vi "_BlankServer.vi"() -> ()   [LabVIEW 2010]
doc: "Template server that runs individual ros topics, services, etc. This is cloned for each topic being run."
uses:
  <userlib>/ROSforLV_0.1/ROS/Code/SubVIs/_ROSControl.ctl
  <userlib>/ROSforLV_0.1/ROS/Code/SubVIs/_ROSDirection.ctl
  <userlib>/ROSforLV_0.1/ROS/Code/_ROSDefinition.vi
panel:
  out "str to write":string
  out "Status":T1(ring) caption="Connected?"
  out "Specs":T3={"Server"="", "Node"="/labview", "Server Port"=5000, "URI (Subsc)"="", "Direction"=enum."Node"}
  out "Service Reply":string
  out "unregister":string="<?xml version='1.0'?>\n<methodResponse>\n<params>\n<param>\n<value><array><data>\n<value><int>1</int></value>\n<value><string>Registered [/labview] as publisher of [/robot/head/command_head_nod]</string></value>\n<value><array><data>\n<value><string>http://tuftsBaxter.local:56995/</string></value>\n</data></array></value>\n</data></array></value>\n</param>\n</params>\n</methodResponse>\n"
  out "Requests":T4(array[cluster])
  out "Last Reply":string
  in  "stop":bool
  out "error out":errorcluster
  out "Connections":T5(array[cluster])
  in  "Baxter":T6
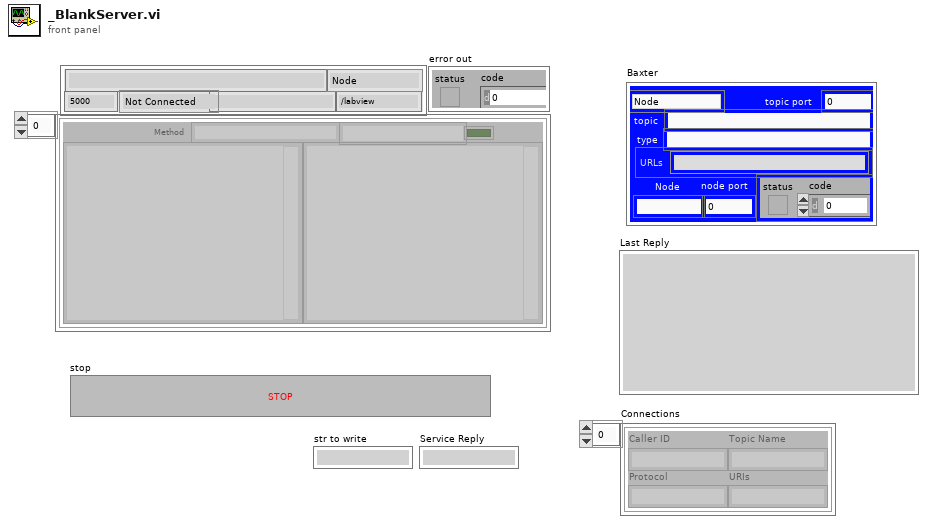
[diagram p1: front panel]
types:
  T1 = enum16{"Not Connected", "Registered", "Connected"}
  T2 = typedef "_ROSDirection.ctl" = enum16{"Node", "Publisher", "Subscriber", "Service Client"}
  T3 = cluster{"Server":string, "Node":string, "Server Port":u32, "URI (Subsc)":string, "Direction":T2}
  T4 = cluster{"First":string, "Second":string, "Method":string, "success":bool, "Dir1":string, "Dir2":string, "time":string}[]
  T5 = cluster{"Caller ID":string, "Topic Name":string, "Protocol":string, "URIs":string}[]
  T6 = typedef "_ROSControl.ctl" = cluster{"topic port":u16, "Node":string, "topic":string, "type":string, "node port":u32, "error ":errorcluster, "Direction":T2, "APIs":string[]}
  T7 = cluster{"data out":string, "data out 2":string, "data out 3":string, "Success?":bool, "data out 4":string, "data out 5":string, "time":string}[]
  T8 = cluster{"Code":i32, "Status Message":string, "APIs":string[]}
  T9 = cluster{"Server":string, "Node":string, "Server Port":u32, "URI (Subsc)":string, "connection":refnum<k5>, "Direction":T2}
  T10 = cluster{"Caller ID":string, "Topic Name":string, "Protocol":string, "URIs":string}
  T11 = cluster{string, "data out":string, "Node":string, bool, string, string, "Current Time":string}
  T12 = cluster{"str to write":string, string, string, bool, string, string, "Current Time":string}
  T13 = cluster{"Protocol":string, "Code":i32, "IP":string, "Port":i32}
  T14 = cluster{"Node":string, "topic":string, "topic":string, "topic":string}
  T15 = cluster{"Code":i8, "statusMessage":string, "APIs":string[]}
  T16 = cluster{string, string, string, bool, string, string, "Current Time":string}
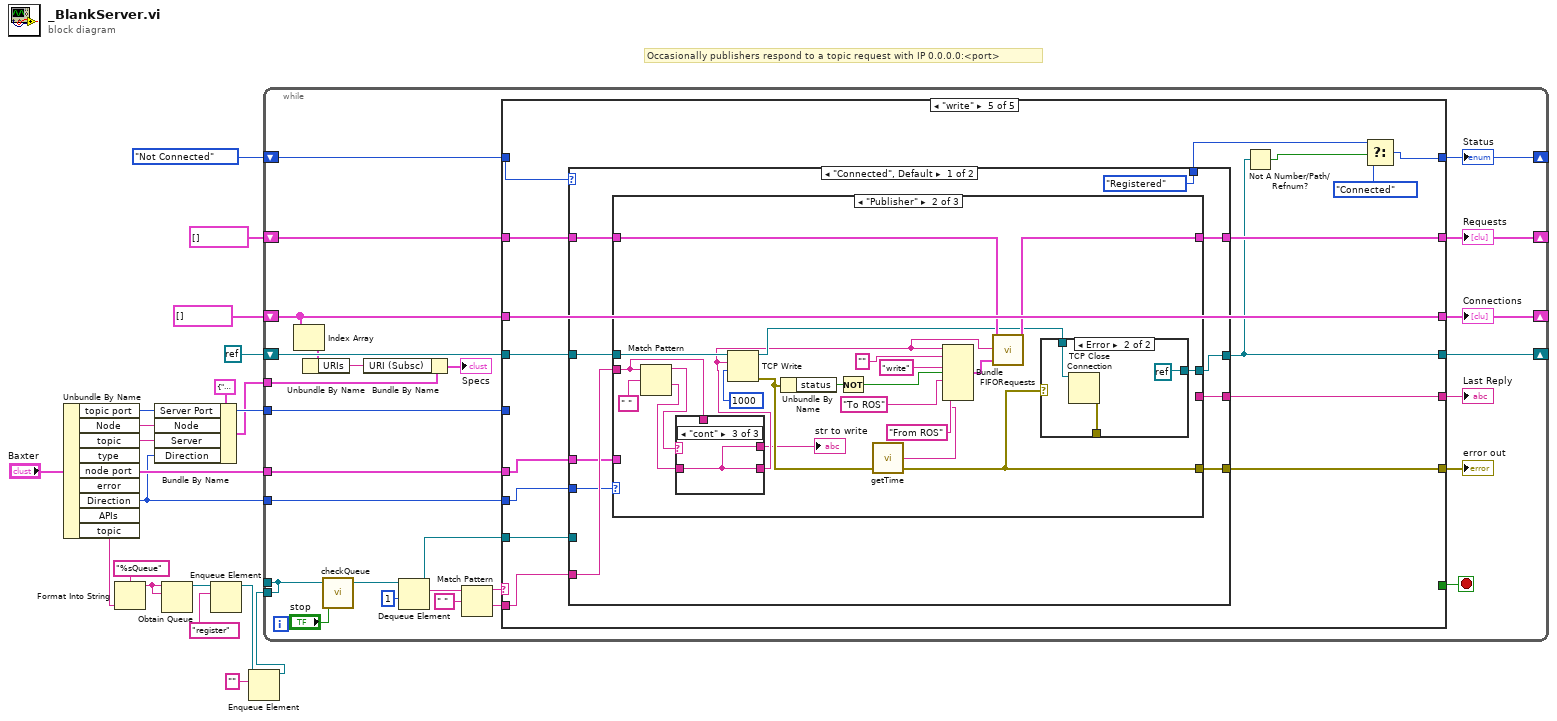
[diagram p0: block diagram]
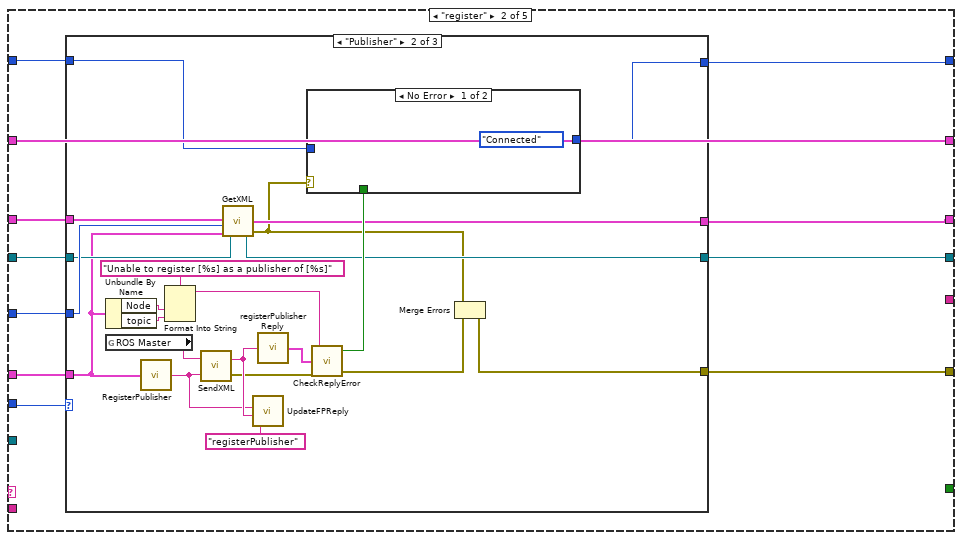
[diagram p3: hidden frame]
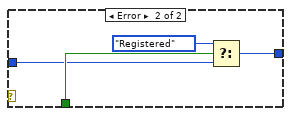
[diagram p5: hidden frame]
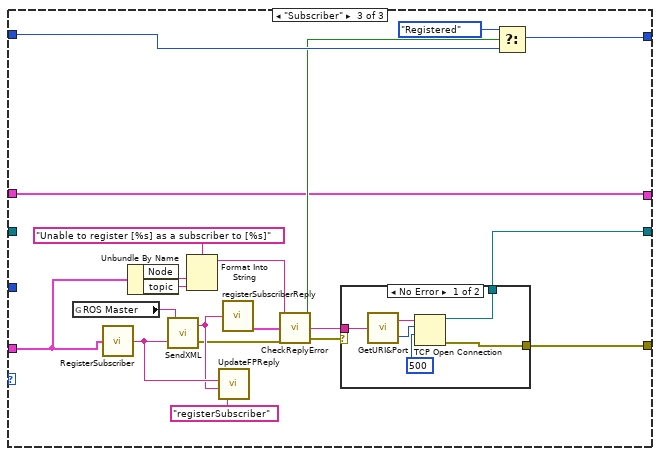
[diagram p6: hidden frame]
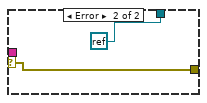
[diagram p7: hidden frame]
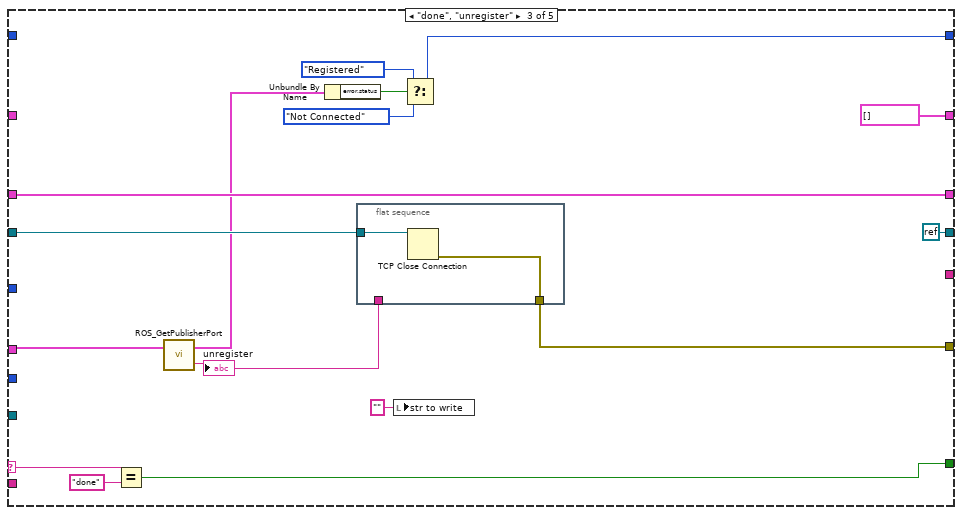
[diagram p8: hidden frame]
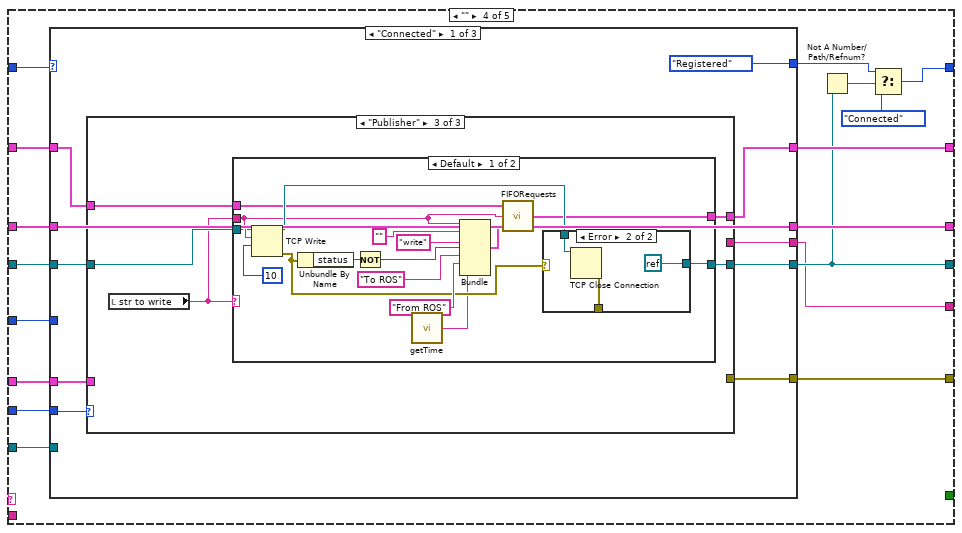
[diagram p9: hidden frame]
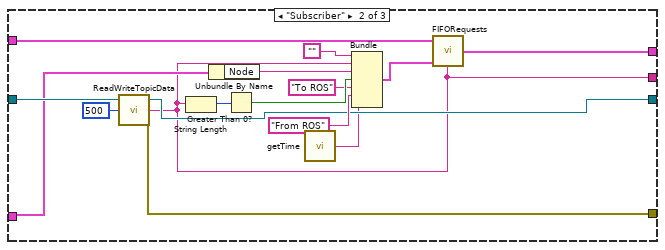
[diagram p11: hidden frame]
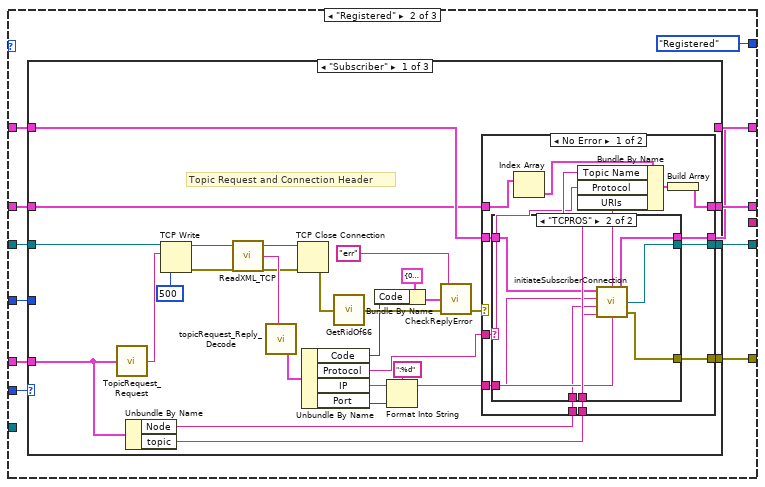
[diagram p14: hidden frame]
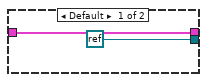
[diagram p15: hidden frame]
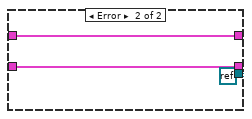
[diagram p16: hidden frame]
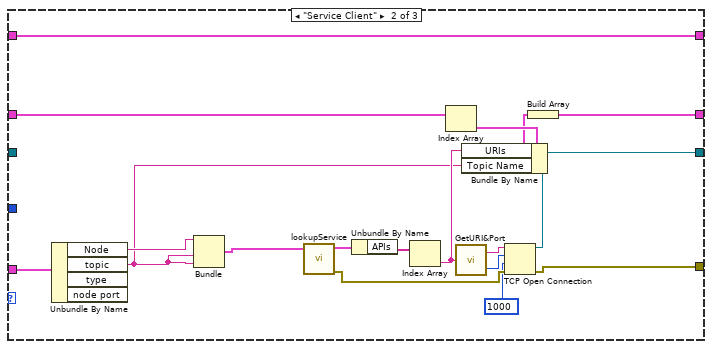
[diagram p17: hidden frame]
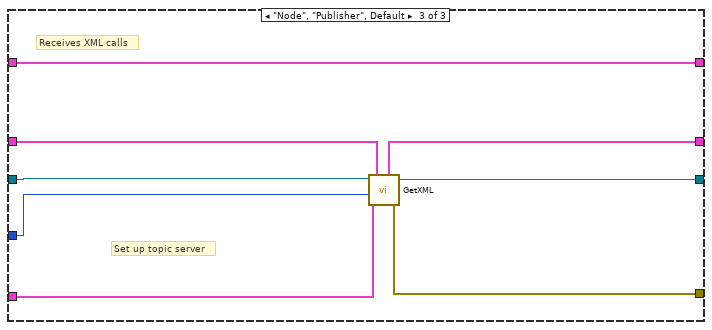
[diagram p18: hidden frame]
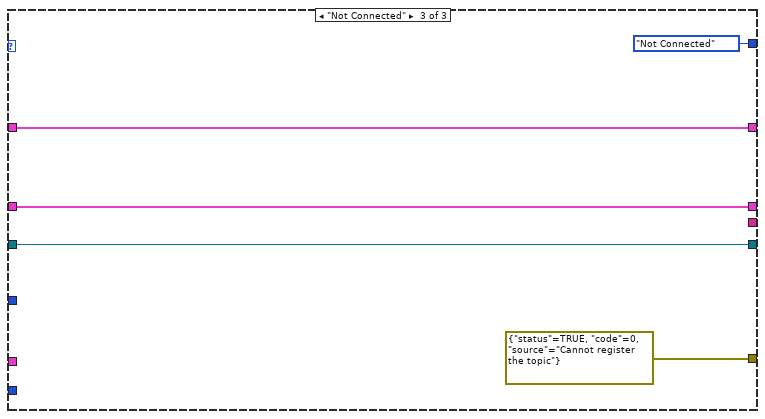
[diagram p19: hidden frame]
diagram:
  # "Occasionally publishers respond to a topic request with IP 0.0.0.0:<port>"
  n1 = Unbundle By Name("Baxter") -> ("topic port"=w10:u16, "Node"=w9:string, "topic"=w8:string, "Direction"=w7:T2, "topic"=w5:string)  [unwired: 4 out]
  n2 = Format Into String(format string="%sQueue", w5) -> (resulting string=w18:string)  [unwired: 2 in, 1 out]
  n3 = Bundle By Name(cluster=T3 {"Server"="", "Node"="/labview", "Server Port"=5000, "URI (Subsc)"="", "Direction"=enum."Node"} ("Specs"), "Server Port"=w10, "Node"=w9, "Server"=w8, "Direction"=w7) -> (w6:T3)
  n4 = Obtain Queue(name (unnamed)=w18, element data type=w18) -> (queue out=w12:refnum<queue>)  [unwired: 3 in, 2 out]
  n5 = Enqueue Element(queue=w12, element="register") -> (queue out=w3:refnum<queue>)  [unwired: 2 in, 2 out]
  n6 = Enqueue Element(queue=w3, element="") -> (queue out=w2:refnum<queue>)  [unwired: 2 in, 2 out]
  n7 = while {
    tunnel: w10 -> [w46]
    shift-right: [w30] -> _
    shift-left: T5 [] ("Connections") -> [w28]
    shift-right: [w35] -> _
    shift-left: refnum<k0> refnum -> [w44]
    tunnel: w7 -> [w45]
    tunnel: "Baxter" -> [w43]
    tunnel: [w20] -> _
    shift-right: [w36] -> _
    shift-left: T7 [] ("Requests In") -> [w37]
    shift-right: [w32] -> _
    shift-left: T1."Not Connected" ("Status") -> [w33]
    tunnel: w6 -> [w26]
    tunnel: w2 -> [w20]
    stop <- w34 stop-if-true
    n8 = Index Array(array=w28) -> (element=w27:T10)  [unwired: 1 in]
    n9 = Unbundle By Name(w27) -> ("URIs"=w25:string)
    n10 = call <userlib>:"checkQueue.vi"("stop"="stop", "queue in"=w20) -> ("queue out"=w22:refnum<queue>)  [unwired: 3 in]
    n11 = Bundle By Name(cluster=w26, "URI (Subsc)"=w25) -> (→"Specs":T3)
    n12 = Dequeue Element(queue=w22, timeout in ms (-1)=1) -> (queue out=w23:refnum<queue>, element=w41:string)  [unwired: 1 in, 2 out]
    n13 = Match Pattern(string=w41, regular expression=" ") -> (before substring=w39:string, after substring=w38:string)  [unwired: 1 in, 2 out]
    n14 = case shown="\"write\"" w39 {
      selector: w39 -> [_ _ w124 _ _]
      tunnel: w46 -> [_ w60 _ w154 _]
      tunnel: w28 -> [w50 w52 w134 w153 w321]
      tunnel: [w50 w51 w134 w152 w321] -> w30
      tunnel: w45 -> [_ w61 _ w151 w313]
      tunnel: [w49 w57 refnum<k0> refnum w145 w314] -> w35
      tunnel: w44 -> [w49 w56 w135 w146 w320]
      tunnel: w43 -> [_ w59 w133 w150 w311]
      tunnel: w38 -> [_ _ _ _ w318]
      tunnel: [_ _ w122 _ _] -> w34
      tunnel: [_ w58 w127 w147 w315] -> w31
      tunnel: w37 -> [w48 w55 _ w149 w317]
      tunnel: [w48 w55 T7 [] ("Requests Out") w148 w316] -> w36
      tunnel: w33 -> [w47 w54 _ w139 w319]
      tunnel: [w47 w53 w129 w140 w306] -> w32
      tunnel: [_ _ _ w144 w312] -> w29
      tunnel: w23 -> [_ _ _ w143 w310]
      frame Default {
      }
      frame "register" {
        n15 = case shown="\"Publisher\"" w61 {
          tunnel: w60 -> [_ w71 _]
          tunnel: w59 -> [_ w68 w102]
          tunnel: [_ w66 w99] -> w58
          tunnel: [w64 w69 w100] -> w57
          tunnel: w56 -> [w64 w70 _]
          tunnel: w54 -> [w63 w75 w95]
          tunnel: [w63 w74 w93] -> w53
          tunnel: w52 -> [w62 w73 w92]
          tunnel: [w62 w72 w92] -> w51
          frame "Node", Default {
          }
          frame "Publisher" {
            n16 = Unbundle By Name(w68) -> ("Node"=w82:string, "topic"=w81:string)
            n17 = global read "_ROSDefinition.vi" "ROS Master"() -> (w86:string)
            n18 = call <userlib>:"RegisterPublisher.vi"("ROS"=w68) -> ("XML"=w80:string)
            n19 = Format Into String(format string="Unable to register [%s] as a publisher of [%s]", w82, w81) -> (resulting string=w78:string)  [unwired: 2 in, 1 out]
            n20 = call <userlib>:"SendXML.vi"("Send"=w80, "URI in"=w86) -> ("error out"=w77:errorcluster, "Reply"=w85:string)
            n21 = call <userlib>:"GetXML.vi"("Baxter"=w68, "topic port"=w71, "Connections"=w73, "connection ID in"=w70) -> ("error IO"=w65:errorcluster, "Subscribers"=w72:T5, "connection ID out"=w69:refnum<k5>)
            n22 = call <userlib>:"UpdateFPReply.vi"("Reply"=w85, "Sent"=w80, "method"="registerPublisher") -> ()  [unwired: 3 in]
            n23 = call <userlib>:"registerPublisherReply.vi"("Response"=w85) -> ("Response"=w79:T8)
            n24 = call <userlib>:"CheckReplyError.vi"("error in"=w77, "Response"=w79, "Error String"=w78) -> ("error out"=w67:errorcluster, "Registered?"=w76:bool)  [unwired: 1 out]
            n25 = case shown="No Error" w65 {
              tunnel: w76 -> [_ w91]
              tunnel: w75 -> [_ w90]
              tunnel: [T1."Connected" ("f") w88] -> w74
              frame No Error {
              }
              frame Error {
                n26 = Select(t=T1."Registered", s=w91, f=w90) -> (s? t:f=w88:T1)
              }
            }
            n27 = Merge Errors(w65, w67) -> (w66:errorcluster)
          }
          frame "Subscriber" {
            n28 = global read "_ROSDefinition.vi" "ROS Master"() -> (w111:string)
            n29 = call <userlib>:"RegisterSubscriber.vi"("ROS"=w102) -> ("XML"=w109:string)
            n30 = Unbundle By Name(w102) -> ("Node"=w106:string, "topic"=w105:string)
            n31 = call <userlib>:"SendXML.vi"("Send"=w109, "URI in"=w111) -> ("error out"=w98:errorcluster, "Reply"=w108:string)
            n32 = Format Into String(format string="Unable to register [%s] as a subscriber to [%s]", w106, w105) -> (resulting string=w103:string)  [unwired: 2 in, 1 out]
            n33 = call <userlib>:"UpdateFPReply.vi"("Reply"=w108, "Sent"=w109, "method"="registerSubscriber") -> ()  [unwired: 3 in]
            n34 = call <userlib>:"registerSubscriberReply.vi"("Response"=w108) -> ("Response"=w107:T8)
            n35 = call <userlib>:"CheckReplyError.vi"("error in"=w98, "Response"=w107, "Error String"=w103) -> ("error out"=w97:errorcluster, "URI"=w101:string, "Registered?"=w94:bool)
            n36 = case shown="No Error" w97 {
              selector: w97 -> [_ w119]
              tunnel: w101 -> [w117 _]
              tunnel: [w113 refnum<k0> refnum] -> w100
              tunnel: [w112 w119] -> w99
              frame No Error {
                n37 = call <userlib>:"GetURI&Port.vi"("URI in"=w117) -> ("Port"=w115:u16, "URI"=w116:string)
                n38 = TCP Open Connection(address=w116, remote port or service name=w115, timeout ms (60000)=500) -> (connection ID=w113:refnum<k5>, error out=w112:errorcluster)  [unwired: 2 in]
              }
              frame Error {
              }
            }
            n39 = Select(t=T1."Registered", s=w94, f=w95) -> (s? t:f=w93:T1)
          }
        }
      }
      frame "done", "unregister" {
        n40 = Equal?(x=w124, y="done") -> (x = y?=w122:bool)
        n41 = call <userlib>:"ROS_GetPublisherPort.vi"("ROS in"=w133) -> ("Response"=w125:string, "ROS out"=w132:T6)  [unwired: 1 in]
        "unregister" <- w125
        n42 = Unbundle By Name(w132) -> ("error.status"=w128:bool)
        n43 = flat-sequence {
          tunnel: w135 -> [w137]
          tunnel: [w136] -> w127
          tunnel: w125 -> [_]
          frame #0 {
            n44 = TCP Close Connection(connection ID=w137) -> (error out=w136:errorcluster)  [unwired: 2 in, 1 out]
          }
        }
        n45 = local write "str to write"("" ("str to write")) -> ()
        n46 = Select(t=T1."Registered" ("Status"), s=w128, f=T1."Not Connected") -> (s? t:f=w129:T1)
      }
      frame "" {
        n47 = case shown="\"Connected\"" w139 {
          tunnel: w154 -> [_ w220 _]
          tunnel: w153 -> [w163 w219 w304]
          tunnel: [w163 w218 w304] -> w152
          tunnel: w151 -> [w164 w217 _]
          tunnel: [w157 w216 w303] -> w145
          tunnel: w146 -> [w162 w215 w303]
          tunnel: w150 -> [w161 w214 _]
          tunnel: w149 -> [w160 w213 w305]
          tunnel: [w159 w212 w305] -> w148
          tunnel: [w158 w211 errorcluster {"status"=TRUE, "code"=0, "source"="Cannot register the topic"} ("error out")] -> w147
          tunnel: [w156 _ _] -> w144
          tunnel: w143 -> [_ _ _]
          tunnel: [T1."Registered" ("f") T1."Registered" ("f") T1."Not Connected" ("f")] -> w138
          frame "Connected" {
            n48 = case shown="\"Publisher\"" w164 {
              tunnel: w162 -> [w165 w182 w185]
              tunnel: w161 -> [_ w175 _]
              tunnel: w160 -> [w166 w180 w187]
              tunnel: [w166 w179 w186] -> w159
              tunnel: [_ w178 _] -> w158
              tunnel: [w165 w169 w184] -> w157
              tunnel: [_ w168 _] -> w156
              frame "Node", Default {
              }
              frame "Subscriber" {
                n49 = call <userlib>:"ReadWriteTopicData.vi"("timeout ms (1000)"=500, "connection ID in"=w182) -> ("error out"=w178:errorcluster, "data out"=w168:string, "connection ID out"=w169:refnum<k5>)  [unwired: 1 in]
                n50 = String Length(string=w168) -> (length=w177:i32)
                n51 = Unbundle By Name(w175) -> ("Node"=w174:string)
                n52 = Greater Than 0?(x=w177) -> (x > 0?=w173:bool)
                n53 = call <userlib>:"getTime.vi"() -> ("Current Time"=w167:string)  [unwired: 1 in]
                n54 = Bundle("", "data out"=w168, "Node"=w174, w173, "To ROS", "From ROS", "Current Time"=w167) -> (w170:T11)  [unwired: 1 in]
                n55 = call <userlib>:"FIFORequests.vi"("New One"=w170, "data out"=w168, "Requests In"=w180) -> ("Requests Out"=w179:T7)
              }
              frame "Publisher" {
                n56 = local read "str to write"() -> (w183:string)
                n57 = case shown="Default" w183 {
                  tunnel: w187 -> [w196 w209]
                  tunnel: [w195 w209] -> w186
                  tunnel: w185 -> [w192 w208]
                  tunnel: [w191 w208] -> w184
                  tunnel: w183 -> [w193 _]
                  frame Default {
                    n58 = TCP Write(connection ID=w192, data in=w193, 9:10 ("timeout ms (25000)")) -> (connection ID out=w197:refnum<k5>, error out=w190:errorcluster)  [unwired: 1 in, 1 out]
                    n59 = Unbundle By Name(w190) -> ("status"=w199:bool)
                    n60 = Not(x=w199) -> (.not. x?=w198:bool)
                    n61 = call <userlib>:"getTime.vi"() -> ("Current Time"=w188:string)  [unwired: 1 in]
                    n62 = Bundle("str to write"=w193, "", "write", w198, "To ROS", "From ROS", "Current Time"=w188) -> (w200:T12)  [unwired: 1 in]
                    n63 = call <userlib>:"FIFORequests.vi"("New One"=w200, "data out"=w193, "Requests In"=w196) -> ("Requests Out"=w195:T7)
                    n64 = case shown="Error" w190 {
                      tunnel: w197 -> [w204 w207]
                      tunnel: [w204 refnum<k0> refnum] -> w191
                      tunnel: [_ w205] -> _
                      frame No Error {
                      }
                      frame Error {
                        n65 = TCP Close Connection(connection ID=w207) -> (error out=w205:errorcluster)  [unwired: 2 in, 1 out]
                      }
                    }
                  }
                  frame "" {
                  }
                }
              }
            }
          }
          frame "Registered" {
            n66 = case shown="\"Subscriber\"" w217 {
              tunnel: w220 -> [_ _ w293]
              tunnel: w219 -> [w229 w280 w300]
              tunnel: [w228 w278 w299] -> w218
              tunnel: [w233 w284 w298] -> w216
              tunnel: w215 -> [w250 _ w294]
              tunnel: w214 -> [w238 w291 w297]
              tunnel: w213 -> [w236 w292 w296]
              tunnel: [w235 w292 w296] -> w212
              tunnel: [w234 w283 w295] -> w211
              frame "Subscriber" {
                # "Topic Request and Connection Header"
                n67 = call <userlib>:"TopicRequest_Request.vi"("ROS"=w238) -> ("XML"=w249:string)
                n68 = Unbundle By Name(w238) -> ("Node"=w237:string, "topic"=w232:string)
                n69 = TCP Write(connection ID=w250, data in=w249, 9:500 ("timeout ms (25000)")) -> (connection ID out=w248:refnum<k5>, error out=w247:errorcluster)  [unwired: 1 in, 1 out]
                n70 = call <userlib>:"ReadXML_TCP.vi"("error in"=w247, "connection ID in"=w248) -> ("error out"=w243:errorcluster, "data out"=w245:string, "connection ID out"=w244:refnum<k5>)  [unwired: 1 in]
                n71 = call <userlib>:"topicRequest_Reply_Decode.vi"("Topic Request Reply"=w245) -> ("Topic Request Reply"=w242:T13)
                n72 = TCP Close Connection(connection ID=w244, error in (no error)=w243) -> (error out=w241:errorcluster)  [unwired: 1 in, 1 out]
                n73 = Unbundle By Name(w242) -> ("Code"=w223:i32, "Protocol"=w231:string, "IP"=w227:string, "Port"=w239:i32)
                n74 = call <userlib>:"GetRidOf66.vi"("error in (no error)"=w241) -> ("error out"=w225:errorcluster)
                n75 = Bundle By Name(cluster=T8 {"Code"=0, "Status Message"="", "APIs"=[]} ("Response"), "Code"=w223) -> (w221:T8)
                n76 = Format Into String(format string=":%d", initial string=w227, w239) -> (resulting string=w230:string)  [unwired: 1 in, 1 out]
                n77 = call <userlib>:"CheckReplyError.vi"("error in"=w225, "Response"=w221, "Error String"="err" ("source")) -> ("error out"=w224:errorcluster)  [unwired: 2 out]
                n78 = case shown="No Error" w224 {
                  tunnel: w231 -> [w254 _]
                  tunnel: w230 -> [w253 _]
                  tunnel: w237 -> [w262 _]
                  tunnel: w232 -> [w255 _]
                  tunnel: w236 -> [w261 w272]
                  tunnel: [w260 w272] -> w235
                  tunnel: [w259 _] -> w234
                  tunnel: [w258 refnum<k0> refnum] -> w233
                  tunnel: w229 -> [w257 w273]
                  tunnel: [w251 w273] -> w228
                  frame No Error {
                    n79 = case shown="\"TCPROS\"" w254 {
                      tunnel: w253 -> [_ w271]
                      tunnel: w262 -> [_ w270]
                      tunnel: w255 -> [_ w269]
                      tunnel: w261 -> [w263 w265]
                      tunnel: [w263 w268] -> w260
                      tunnel: [_ w267] -> w259
                      tunnel: [refnum<k0> refnum w266] -> w258
                      frame Default {
                      }
                      frame "TCPROS" {
                        n80 = call <userlib>:"initiateSubscriberConnection.vi"("topic"=w269, "Node"=w270, "URI"=w271, "Requests In"=w265) -> ("error out"=w267:errorcluster, "connection ID out"=w266:refnum<k5>, "Requests Out"=w268:T7)
                      }
                    }
                    n81 = Index Array(array=w257) -> (element=w256:T10)  [unwired: 1 in]
                    n82 = Bundle By Name(cluster=w256, "Topic Name"=w255, "Protocol"=w254, "URIs"=w253) -> (w252:T10)
                    n83 = Build Array(w252) -> (w251:T5)
                  }
                  frame Error {
                  }
                }
              }
              frame "Service Client" {
                n84 = Unbundle By Name(w291) -> ("Node"=w290:string, "topic"=w276:string)  [unwired: 2 out]
                n85 = Bundle("Node"=w290, "topic"=w276, "topic"=w276, "topic"=w276) -> (w289:T14)  [unwired: 1 in]
                n86 = call <userlib>:"lookupService.vi"("Parameters"=w289) -> ("Reply"=w288:T15, "error out"=w277:errorcluster)  [unwired: 4 in, 2 out]
                n87 = Unbundle By Name(w288) -> ("APIs"=w287:string[])
                n88 = Index Array(array=w287) -> (element=w281:string)  [unwired: 1 in]
                n89 = Index Array(array=w280) -> (element=w282:T10)  [unwired: 1 in]
                n90 = call <userlib>:"GetURI&Port.vi"("URI in"=w281) -> ("Port"=w285:u16, "URI"=w286:string)
                n91 = Bundle By Name(cluster=w282, "URIs"=w281, "Topic Name"=w276) -> (w279:T10)
                n92 = TCP Open Connection(address=w286, remote port or service name=w285, timeout ms (60000)=1000, error in (no error)=w277) -> (connection ID=w284:refnum<k5>, error out=w283:errorcluster)  [unwired: 1 in]
                n93 = Build Array(w279) -> (w278:T5)
              }
              frame "Node", "Publisher", Default {
                # "Set up topic server"
                # "Receives XML calls"
                n94 = call <userlib>:"GetXML.vi"("Baxter"=w297, "topic port"=w293, "Connections"=w300, "connection ID in"=w294) -> ("error IO"=w295:errorcluster, "Subscribers"=w299:T5, "connection ID out"=w298:refnum<k5>)
              }
            }
          }
          frame "Not Connected" {
          }
        }
        n95 = Not A Number/Path/Refnum?(number/path/refnum=w145) -> (NaN/Path/Refnum?=w141:bool)
        n96 = Select(t=w138, s=w141, f=T1."Connected") -> (s? t:f=w140:T1)
      }
      frame "write" {
        n97 = case shown="\"Connected\", Default" w319 {
          tunnel: w320 -> [w331 w385]
          tunnel: w318 -> [w328 w382]
          tunnel: w317 -> [w330 w386]
          tunnel: [w329 w386] -> w316
          tunnel: [w326 w385] -> w314
          tunnel: [w327 _] -> w315
          tunnel: w313 -> [w325 _]
          tunnel: [w324 _] -> w312
          tunnel: w311 -> [w323 _]
          tunnel: w310 -> [_ w384]
          tunnel: [T1."Registered" ("f") T1."Connected" ("f")] -> w307
          frame "Connected", Default {
            n98 = case shown="\"Publisher\"" w325 {
              tunnel: w331 -> [w332 w354 w370]
              tunnel: w330 -> [w333 w352 w379]
              tunnel: [w333 w351 w378] -> w329
              tunnel: w328 -> [_ w335 w377]
              tunnel: [_ w343 w376] -> w327
              tunnel: [w332 w341 refnum<k0> refnum] -> w326
              tunnel: [_ _ w375] -> w324
              tunnel: w323 -> [_ _ w374]
              frame "Node", Default {
              }
              frame "Publisher" {
                n99 = Match Pattern(string=w335, regular expression=" ") -> (before substring=w336:string, after substring=w337:string)  [unwired: 1 in, 2 out]
                n100 = case shown="\"cont\"" w336 {
                  tunnel: w337 -> [_ w358 w359]
                  tunnel: [w355 w358 w359] -> w339
                  tunnel: ["" "" w359] -> w338
                  tunnel: w335 -> [w355 _ _]
                  frame Default {
                  }
                  frame "stop_cont" {
                  }
                  frame "cont" {
                  }
                }
                "str to write" <- w338
                n101 = TCP Write(connection ID=w354, data in=w339, 9:1000 ("timeout ms (25000)")) -> (connection ID out=w342:refnum<k5>, error out=w343:errorcluster)  [unwired: 1 in, 1 out]
                n102 = Unbundle By Name(w343) -> ("status"=w345:bool)
                n103 = Not(x=w345) -> (.not. x?=w344:bool)
                n104 = call <userlib>:"getTime.vi"() -> ("Current Time"=w334:string)  [unwired: 1 in]
                n105 = Bundle(w339, "", "write", w344, "To ROS", "From ROS", "Current Time"=w334) -> (w346:T16)  [unwired: 1 in]
                n106 = call <userlib>:"FIFORequests.vi"("New One"=w346, "data out"=w339, "Requests In"=w352) -> ("Requests Out"=w351:T7)
                n107 = case shown="Error" w343 {
                  tunnel: w342 -> [w360 w363]
                  tunnel: [w360 refnum<k0> refnum] -> w341
                  tunnel: [_ w361] -> _
                  frame No Error {
                  }
                  frame Error {
                    n108 = TCP Close Connection(connection ID=w363) -> (error out=w361:errorcluster)  [unwired: 2 in, 1 out]
                  }
                }
              }
              frame "Service Client" {
                n109 = Unbundle By Name(w374) -> ("topic"=w366:string, "Node"=w367:string, "APIs"=w372:string[], "Direction"=w365:T2)
                n110 = Index Array(array=w372) -> (element=w371:string)  [unwired: 1 in]
                n111 = local write "Service Reply"("" ("Service Reply")) -> ()
                n112 = Bundle By Name(cluster=T9 {"Server"="", "Node"="/labview", "Server Port"=5000, "URI (Subsc)"="", "connection"=refnum, "Direction"=enum."Node"} ("Specs"), "Server"=w366, "Node"=w367, "URI (Subsc)"=w371, "connection"=w370, "Direction"=w365) -> (w369:T9)
                n113 = call <userlib>:"ROS_Service_Setup.vi"("Specs"=w369, "Msg to Send"=w377, "Requests In"=w379) -> ("error out"=w376:errorcluster, "Reply"=w375:string, "Requests Out"=w378:T7)
                "Service Reply" <- w375
              }
            }
          }
          frame "Not Connected" {
            n114 = Format Into String(format string="write %s", w382) -> (resulting string=w381:string)  [unwired: 2 in, 1 out]
            n115 = call <userlib>:"cleanQueue.vi"("String"=w381, "queue in"=w384) -> ()  [unwired: 1 in, 1 out]
          }
        }
        n116 = Not A Number/Path/Refnum?(number/path/refnum=w314) -> (NaN/Path/Refnum?=w308:bool)
        n117 = Select(t=w307, s=w308, f=T1."Connected") -> (s? t:f=w306:T1)
      }
    }
    "error out" <- w31
    "Requests" <- w36
    "Status" <- w32
    "Connections" <- w30
    "Last Reply" <- w29
  }
